vi "AnalyzeEvent_Double.vi"(6 "Max triggers?":bool, 9 "Channel - Current":u32, 10 "Channel - Previous":u32, 11 "Is Coincidence?":bool) -> (0 "Coincidence Type":string, 3 "Analyze?":bool)   [LabVIEW 2023]
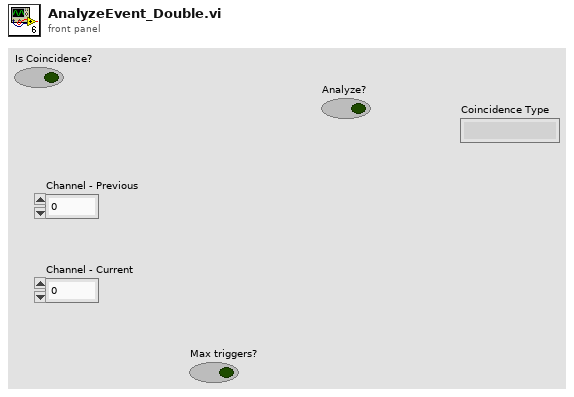
[diagram p1: front panel]
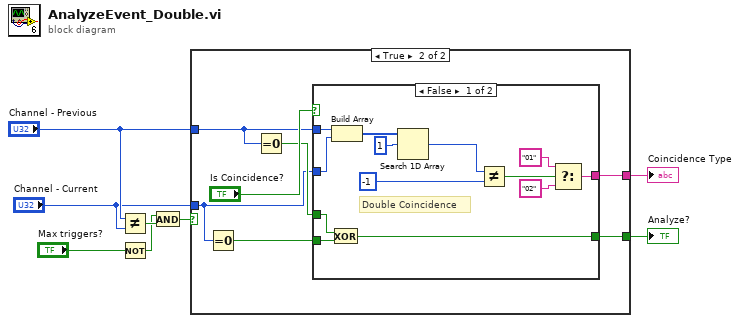
[diagram p0: block diagram]
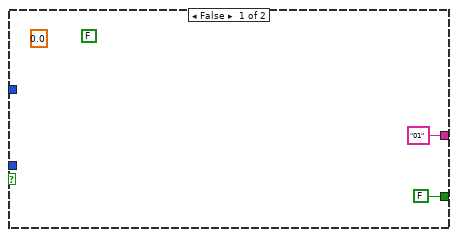
[diagram p2: hidden frame]
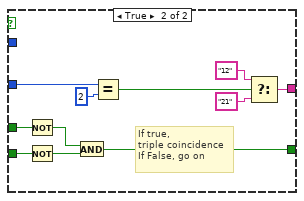
[diagram p3: hidden frame]
diagram:
  n1 = Not Equal?(x="Channel - Previous", y="Channel - Current") -> (x != y?=w8:bool)
  n2 = Not(x="Max triggers?") -> (.not. x?=w1:bool)
  n3 = And(x=w1, y=w8) -> (x .and. y?=w7:bool)
  n4 = case shown="True" w7 {
    tunnel: "Channel - Previous" -> [_ w12]
    tunnel: "Channel - Current" -> [_ w13]
    tunnel: [FALSE w14] -> w4
    tunnel: ["01" ("f") w11] -> w3
    frame False {
      (unwired) 0.0 ("Delay02")
      (unwired) FALSE ("f")
    }
    frame True {
      n5 = Equal To 0?(x=w13) -> (x = 0?=w15:bool)
      n6 = Equal To 0?(x=w12) -> (x = 0?=w16:bool)
      n7 = case shown="False" "Is Coincidence?" {
        tunnel: w16 -> [w30 w41]
        tunnel: w15 -> [w29 w40]
        tunnel: [w28 w38] -> w14
        tunnel: w13 -> [w26 w36]
        tunnel: w12 -> [w27 _]
        tunnel: [w18 w31] -> w11
        frame False {
          # "Double Coincidence"
          n8 = Exclusive Or(1:w29, 2:w30) -> (0:w28:bool)
          n9 = Build Array(w27, w26) -> (w25:u32[])
          n10 = Search 1D Array(1D array=w25, element=u32 1) -> (index of element=w23:i32)  [unwired: 1 in]
          n11 = Not Equal?(x=w23, y=-1) -> (x != y?=w21:bool)
          n12 = Select(t="01", s=w21, f="02") -> (s? t:f=w18:string)
        }
        frame True {
          # "If true,\ntriple coincidence\nIf False, go on"
          n13 = Not(x=w41) -> (.not. x?=w39:bool)
          n14 = Not(x=w40) -> (.not. x?=w37:bool)
          n15 = And(x=w39, y=w37) -> (x .and. y?=w38:bool)
          n16 = Equal?(x=w36, y=u32 2) -> (x = y?=w34:bool)
          n17 = Select(t="12" ("f"), s=w34, f="21") -> (s? t:f=w31:string)
        }
      }
    }
  }
  "Analyze?" <- w4
  "Coincidence Type" <- w3
